vi "setWavelenght.vi"(7 "String":string="setWavelength", 8 "error in (no error)":errorcluster, 11 "wavelength":dbl) -> (0 "error out":errorcluster)   [LabVIEW 2018]
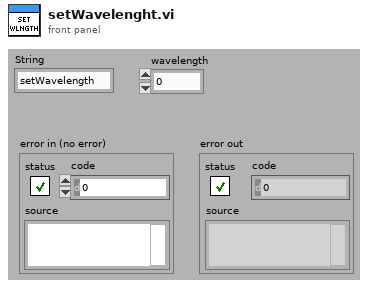
[diagram p1: front panel]
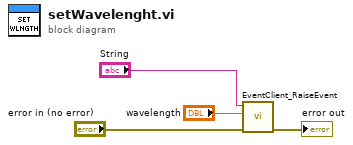
[diagram p0: block diagram]
diagram:
  n1 = call "EventClient_RaiseEvent.vi"("error in (no error)"="error in (no error)", "Data"="wavelength", "Event"="String") -> ("error out"=→"error out":errorcluster)  [unwired: 8 in]
